vi "Sensor_Reads.vi"   [LabVIEW 2019]
uses:
  Globals/Drive_Globals.vi
  <vilib>/Rock Robotics/WPI/ThirdParty/Phoenix-LabVIEW/Motor Controller/Get/CTRE_Phoenix_MotorController_GetSelectedSensorData.vi
  Globals/Sensor_Values.vi
  Globals/Flywheel_Globals.vi
  Globals/Magazine_Globals.vi
  Globals/Control_Panel_Globals.vi
  Globals/Turret_Globals.vi
types:
  T1 = typedef "WPI_MotorControlDeviceRef.ctl" = cluster{"DeviceStatus":errorcluster, "Type":T2, "PWM":cluster{"PWM Channel":T3, "DeadBand":T4}, "CAN":cluster{"Device Number":u8, "SetOutput VI Ref":variant, "GetOutput VI Ref":variant, "Enable VI Ref":variant, "Disable VI Ref":variant, "Data":variant}, "Invert":bool, "DIO PWM":cluster{"PWM \"Enable\" Channel":T3, "DIOChannel":T5, "PWM Rate":dbl}}
  T2 = typedef "WPI_MotorControlType.ctl" = enum16{"PWM", "CAN", "DIO PWM"}
  T3 = typedef "FPGA_DIOPWMChannel.ctl" = enum8{"PWM 0", "PWM 1", "PWM 2", "PWM 3", "PWM 4", "PWM 5", "PWM 6", "PWM 7", "PWM 8", "PWM 9", "PWM MXP 0", "PWM MXP 1", "PWM MXP 2", "PWM MXP 3", "PWM MXP 4", "PWM MXP 5", "PWM MXP 6", "PWM MXP 7", "PWM MXP 8", "PWM MXP 9", "Invalid"}
  T4 = typedef "WPI_PWMDeadband.ctl" = cluster{"Name":string, "maxPositivePwm":i32, "minPositivePwm":i32, "centerPwm":i32, "maxNegativePwm":i32, "minNegativePwm":i32, "angularRange":u16}
  T5 = typedef "FPGA_DIOChannel.ctl" = enum8{"DIO 0", "DIO 1", "DIO 2", "DIO 3", "DIO 4", "DIO 5", "DIO 6", "DIO 7", "DIO 8", "DIO 9", "DIO MXP 0", "DIO MXP 1", "DIO MXP 2", "DIO MXP 3", "DIO MXP 4", "DIO MXP 5", "DIO MXP 6", "DIO MXP 7", "DIO MXP 8", "DIO MXP 9", "DIO MXP 10", "DIO MXP 11", "DIO MXP 12", "DIO MXP 13", "DIO MXP 14", "DIO MXP 15", "SPI Port CS1", "SPI Port CS2", "SPI Port CS3", "SPI Port MISO", "SPI Port MOSI", "Invalid"}
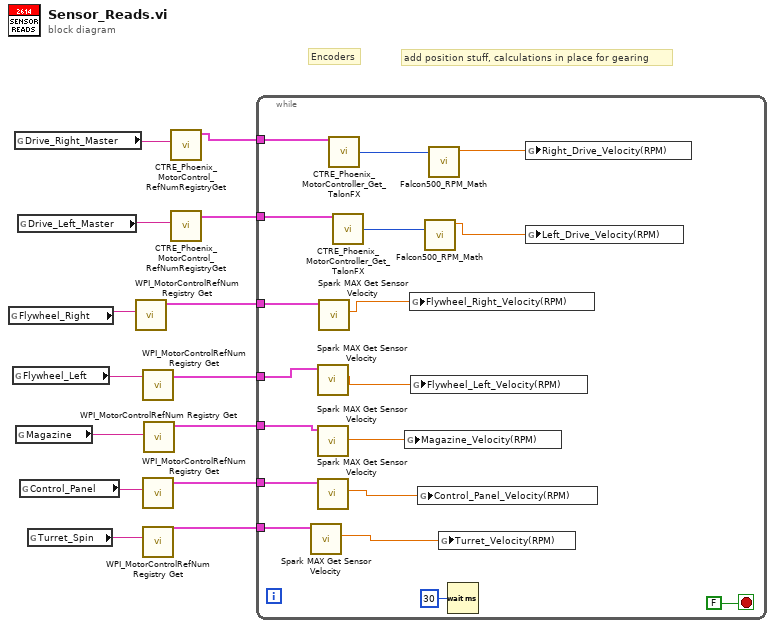
[diagram p0: block diagram]
diagram:
  # "add position stuff, calculations in place for gearing"
  # "Encoders"
  n1 = global read "Flywheel_Globals.vi" "Flywheel_Right"() -> (w9:string)
  n2 = global read "Flywheel_Globals.vi" "Flywheel_Left"() -> (w10:string)
  n3 = global read "Drive_Globals.vi" "Drive_Right_Master"() -> (w13:string)
  n4 = global read "Magazine_Globals.vi" "Magazine"() -> (w6:string)
  n5 = global read "Drive_Globals.vi" "Drive_Left_Master"() -> (w14:string)
  n6 = global read "Control_Panel_Globals.vi" "Control_Panel"() -> (w4:string)
  n7 = global read "Turret_Globals.vi" "Turret_Spin"() -> (w2:string)
  n8 = call <vilib>:"WPI_MotorControlRefNum Registry Get.vi"("refnum name"=w9) -> ("MotorControlDevRef"=w7:T1)  [unwired: 9 in, 1 out]
  n9 = call <vilib>:"WPI_MotorControlRefNum Registry Get.vi"("refnum name"=w10) -> ("MotorControlDevRef"=w8:T1)  [unwired: 9 in, 1 out]
  n10 = call <vilib>:"WPI_MotorControlRefNum Registry Get.vi"("refnum name"=w4) -> ("MotorControlDevRef"=w3:T1)  [unwired: 9 in, 1 out]
  n11 = call <vilib>:"WPI_MotorControlRefNum Registry Get.vi"("refnum name"=w2) -> ("MotorControlDevRef"=w1:T1)  [unwired: 9 in, 1 out]
  n12 = call <vilib>:"WPI_MotorControlRefNum Registry Get.vi"("refnum name"=w6) -> ("MotorControlDevRef"=w5:T1)  [unwired: 9 in, 1 out]
  n13 = call <vilib>:"CTRE_Phoenix_MotorControl_RefNumRegistryGet.vi"("refnum name"=w13) -> ("PhoenixMotorControlDevRef"=w12:T1)  [unwired: 9 in, 1 out]
  n14 = call <vilib>:"CTRE_Phoenix_MotorControl_RefNumRegistryGet.vi"("refnum name"=w14) -> ("PhoenixMotorControlDevRef"=w11:T1)  [unwired: 9 in, 1 out]
  n15 = while {
    tunnel: w12 -> [w31]
    tunnel: w11 -> [w30]
    tunnel: w8 -> [w24]
    tunnel: w7 -> [w23]
    tunnel: w5 -> [w19]
    tunnel: w3 -> [w18]
    tunnel: w1 -> [w16]
    stop <- FALSE stop-if-true
    n16 = call <vilib>:"Spark MAX Get Sensor Velocity.vi"("MotorControlDevRef in"=w16) -> ("Sensor Velocity"=w15:dbl)  [unwired: 7 in, 3 out]
    n17 = call <vilib>:"Spark MAX Get Sensor Velocity.vi"("MotorControlDevRef in"=w24) -> ("Sensor Velocity"=w21:dbl)  [unwired: 7 in, 3 out]
    n18 = call <vilib>:"Spark MAX Get Sensor Velocity.vi"("MotorControlDevRef in"=w19) -> ("Sensor Velocity"=w20:dbl)  [unwired: 7 in, 3 out]
    n19 = call <vilib>:"Spark MAX Get Sensor Velocity.vi"("MotorControlDevRef in"=w18) -> ("Sensor Velocity"=w17:dbl)  [unwired: 7 in, 3 out]
    n20 = call <vilib>:"Spark MAX Get Sensor Velocity.vi"("MotorControlDevRef in"=w23) -> ("Sensor Velocity"=w22:dbl)  [unwired: 7 in, 3 out]
    n21 = call-poly <vilib>:"CTRE_Phoenix_MotorController_Get_TalonFX.vi"("PhoenixMotorControlDevRef"=w31) -> ("Velocity (Raw Sensor Units per 100 ms)"=w29:i32)  [unwired: 11 in, 3 out]
    n22 = call-poly <vilib>:"CTRE_Phoenix_MotorController_Get_TalonFX.vi"("PhoenixMotorControlDevRef"=w30) -> ("Velocity (Raw Sensor Units per 100 ms)"=w27:i32)  [unwired: 11 in, 3 out]
    n23 = global write "Sensor_Values.vi" "Magazine_Velocity(RPM)"(w20) -> ()
    n24 = global write "Sensor_Values.vi" "Flywheel_Right_Velocity(RPM)"(w22) -> ()
    n25 = global write "Sensor_Values.vi" "Flywheel_Left_Velocity(RPM)"(w21) -> ()
    n26 = global write "Sensor_Values.vi" "Control_Panel_Velocity(RPM)"(w17) -> ()
    n27 = call "Falcon500_RPM_Math.vi"("Velocity(native)"=w27) -> ("RPM"=w26:dbl)  [unwired: 10 in]
    n28 = call "Falcon500_RPM_Math.vi"("Velocity(native)"=w29) -> ("RPM"=w28:dbl)  [unwired: 10 in]
    n29 = global write "Sensor_Values.vi" "Turret_Velocity(RPM)"(w15) -> ()
    n30 = Wait (ms)(milliseconds to wait=u32 30) -> ()  [unwired: 1 out]
    n31 = global write "Sensor_Values.vi" "Right_Drive_Velocity(RPM)"(w28) -> ()
    n32 = global write "Sensor_Values.vi" "Left_Drive_Velocity(RPM)"(w26) -> ()
  }
